vi "for_v0_v41.vi"() -> ()   [LabVIEW 2009]
uses:
  <vilib>/Math Plots/3D Math Plots/3D Surface/3D Surface XCtrl/3D Surface.xctl
  <vilib>/Math Plots/3D Math Plots/3D Surface/3D Surface Datatype/3D Surface Datatype.lvclass
  <vilib>/Math Plots/3D Math Plots/3D Surface/3D Surface Datatype/Public/Plot Helper (Vector).vi
  <vilib>/Analysis/Matrix/Numeric/Conversions/Array To Matrix - RA2.vi
  <vilib>/Analysis/Matrix/NI_Matrix.lvlib
panel:
  in  "stop":bool
  in  "Rezolutia":dbl(slide)=36.13636363636363 scale=10.0..100.0
  out "y":dbl=2.000000000000001
  out "X":dbl=2.000000000000001
  out "3D Surface":refnum<class "3D Plot Datatype.lvclass">[](xcontrol)
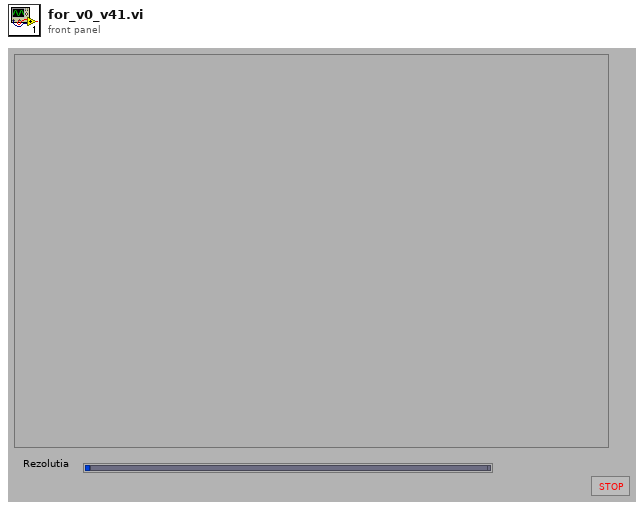
[diagram p1: front panel]
types:
  T1 = typedef "NI_Matrix.lvlib/RealMatrix.ctl" = dbl[][]
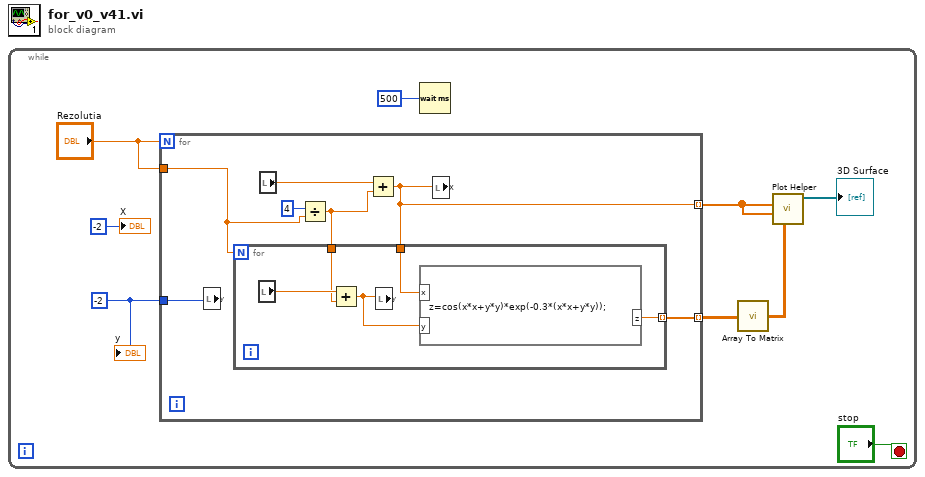
[diagram p0: block diagram]
diagram:
  n1 = while {
    stop <- "stop" stop-if-true
    w3 = -2
    n2 = for {
      N: "Rezolutia" -> [_]
      tunnel: [w15] -> w5 mode=indexing
      tunnel: [w14] -> w6 mode=indexing
      tunnel: "Rezolutia" -> [w12]
      tunnel: w3 -> [w10]
      n3 = local write "y"(w10) -> ()
      n4 = local read "X"() -> (w16:dbl)
      n5 = Divide(x=4, y=w12) -> (x/y=w11:dbl)
      n6 = Add(x=w16, y=w11) -> (x+y=w15:dbl)
      n7 = for {
        N: w12 -> [_]
        tunnel: w15 -> [w20]
        tunnel: [w18] -> w14 mode=indexing
        tunnel: w11 -> [w17]
        n8 = local read "y"() -> (w21:dbl)
        n9 = Add(x=w21, y=w17) -> (x+y=w19:dbl)
        n10 = local write "y"(w19) -> ()
        n11 = formula code="z=cos(x*x+y*y)*exp(-0.3*(x*x+y*y));"("x"=w20, "y"=w19) -> ("z"=w18:dbl)
      }
      n12 = local write "X"(w15) -> ()
    }
    n13 = Wait (ms)(milliseconds to wait=500) -> ()  [unwired: 1 out]
    n14 = call-poly <vilib>:"Array To Matrix.vi"("Real 2D Array"=w6) -> ("Real Matrix"=w7:T1)
    n15 = call-poly <vilib>:"Plot Helper.vi"("z matrix"=w7, "y vector"=w5, "x vector"=w5) -> ("3D Plot lvclass Array out"=→"3D Surface":refnum<class "3D Plot Datatype.lvclass">[])  [unwired: 3 in, 5 out]
    "X" <- -2
    "y" <- w3
  }
